vi "ProdaNG.Example.SetTV.vi"() -> ()   [LabVIEW 2015]
uses:
  Controls/ProdaNG.Identification.ctl
  Controls/ProdaNG.TestValue.ctl
panel:
  out "TestValue out":T1 {"minimum" format="%#.3f"; "maximum" format="%#.3f"}
  in  "limit":dbl
  out "TV1 2":T1 {"minimum" format="%#.3f"; "maximum" format="%#.3f"}
  out "TV1":T1 {"minimum" format="%#.3f"; "maximum" format="%#.3f"}
  out "IDs":T2
  out "error out":errorcluster {"code" format="%.2f"}
  in  "Connection string":string="szupienko/siemano@proda_wpl_dev"
  in  "System":string="MTB12"
  in  "Wabco Number":string="4611061027"
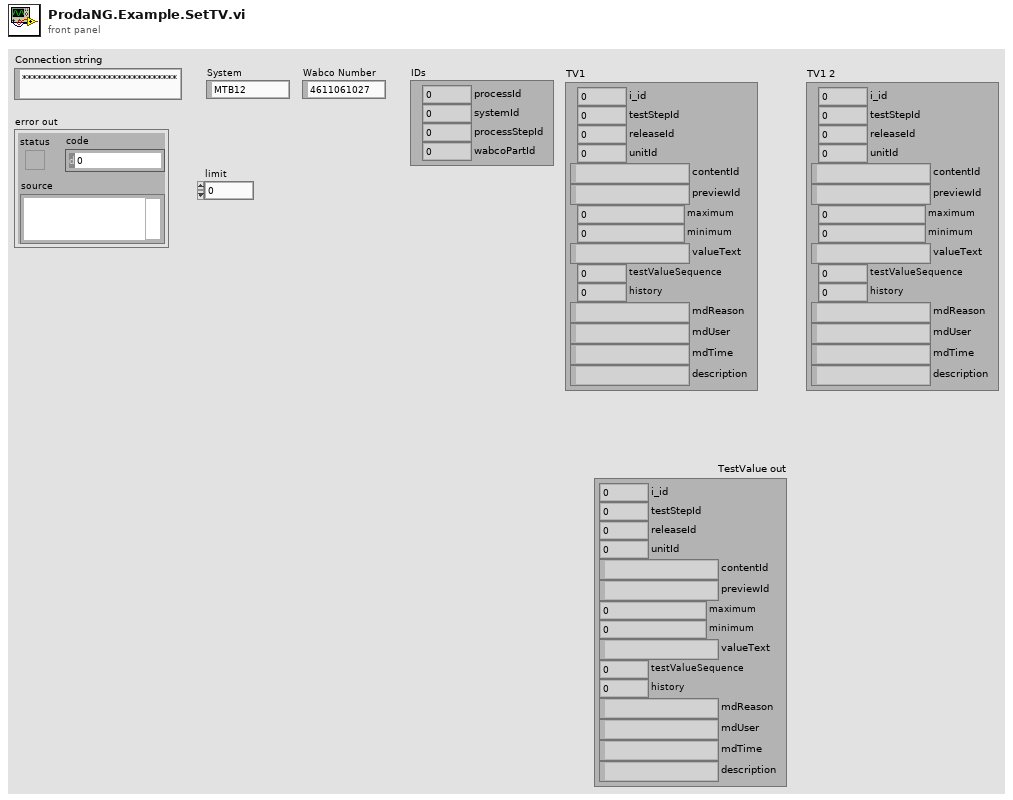
[diagram p1: front panel]
types:
  T1 = typedef "ProdaNG.TestValue.ctl" = cluster{"i_id":i32, "testStepId":i32, "releaseId":i32, "unitId":i32, "contentId":string, "previewId":string, "maximum":dbl, "minimum":dbl, "valueText":string, "testValueSequence":i32, "history":i32, "mdReason":string, "mdUser":string, "mdTime":string, "description":string}
  T2 = typedef "ProdaNG.Identification.ctl" = cluster{"processId":i32, "systemId":i32, "processStepId":i32, "wabcoPartId":i32}
  T3 = typedef "ProdaNG.ProcessStep.ctl" = cluster{"i_id":i32, "processId":i32, "systemId":i32, "releaseId":i32, "processSequence":i32, "limitYellow":dbl, "limitRed":dbl, "mdReason":string, "mdUser":string, "mdTime":string, "filename":string, "transfer":string, "description":string}
  T4 = typedef "ProdaNG.TestStep.ctl" = cluster{"i_id":i32, "processStepId":i32, "testSequence":i32, "testOrder":i32, "mdReason":string, "mdUser":string, "mdTime":string, "description":string}
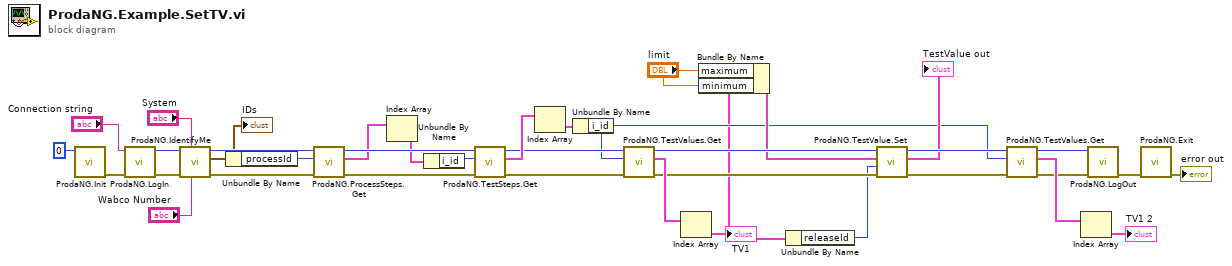
[diagram p0: block diagram]
diagram:
  n1 = call "ProdaNG.Init.vi"("numContexts (0: unlimited)"=0 ("numContexts")) -> ("error out"=w37:errorcluster)  [unwired: 10 in]
  n2 = call "ProdaNG.LogIn.vi"("error in"=w37, "ConnectionString"="Connection string") -> ("error out"=w29:errorcluster, "dbHandle"=w30:i32)  [unwired: 7 in, 1 out]
  n3 = call "ProdaNG.IdentifyMe.vi"("wabcoNumber"="Wabco Number", "systemName"="System", "error in"=w29, "dbHandleIn"=w30) -> ("error out"=w26:errorcluster, "Identification"=w20:T2, "dbHandle"=w28:i32)  [unwired: 5 in]
  "IDs" <- w20
  n4 = Unbundle By Name(w20) -> ("processId"=w24:i32)
  n5 = call "ProdaNG.ProcessSteps.Get.vi"("error in (no error)"=w26, "processId"=w24, "dbHandleIn"=w28) -> ("error out"=w25:errorcluster, "ProcSteps"=w22:T3[], "dbHandle"=w27:i32)  [unwired: 6 in]
  n6 = Index Array(array=w22) -> (element=w19:T3)  [unwired: 1 in]
  n7 = Unbundle By Name(w19) -> ("i_id"=w23:i32)
  n8 = call "ProdaNG.TestSteps.Get.vi"("error in (no error)"=w25, "processStepId"=w23, "dbHandleIn"=w27) -> ("error out"=w16:errorcluster, "TestSteps"=w21:T4[], "dbHandle"=w17:i32)  [unwired: 6 in]
  n9 = Index Array(array=w21) -> (element=w18:T4)  [unwired: 1 in]
  n10 = Unbundle By Name(w18) -> ("i_id"=w6:i32)
  n11 = call "ProdaNG.TestValues.Get.vi"("error in (no error)"=w16, "testStepId"=w6, "dbHandleIn"=w17) -> ("error out"=w13:errorcluster, "TestStepValues"=w15:T1[], "dbHandle"=w14:i32)  [unwired: 6 in]
  n12 = Index Array(array=w15) -> (element=w2:T1)  [unwired: 1 in]
  "TV1" <- w2
  n13 = Bundle By Name(cluster=w2, "maximum"="limit", "minimum"="limit") -> (w9:T1)
  n14 = Unbundle By Name(w2) -> ("releaseId"=w1:i32)
  n15 = call "ProdaNG.TestValue.Set.vi"("error in (no error)"=w13, "ReleaseId"=w1, "TestValue"=w9, "dbHandleIn"=w14) -> ("error out"=w11:errorcluster, "TestValue out"=→"TestValue out":T1, "dbHandle"=w12:i32)  [unwired: 5 in]
  n16 = call "ProdaNG.TestValues.Get.vi"("error in (no error)"=w11, "testStepId"=w6, "dbHandleIn"=w12) -> ("error out"=w4:errorcluster, "TestStepValues"=w5:T1[], "dbHandle"=w3:i32)  [unwired: 6 in]
  n17 = Index Array(array=w5) -> (element=→"TV1 2":T1)  [unwired: 1 in]
  n18 = call "ProdaNG.LogOut.vi"("error in"=w4, "dbHandleIn"=w3) -> ("error out"=w32:errorcluster)  [unwired: 9 in]
  n19 = call "ProdaNG.Exit.vi"("error in (no error)"=w32) -> ("error out"=→"error out":errorcluster)  [unwired: 10 in]
